vi "Fix merge.vi"(8 "error in (no error)":errorcluster, 11 "Control-Client in":refnum<class "Control-Client.lvclass">) -> (0 "error out":errorcluster, 3 "Control-Client out":refnum<class "Control-Client.lvclass">)   [LabVIEW 2019, in "Control-Client.lvclass"]
uses:
  Control-Client.lvclass
  Experiments/Experiment_merged/Experiment_merged.lvclass
  C:/Dev/TRANCON/Classes/Experiments/Experiment.lvclass
  Control-Client.lvclass/Control-Client.ctl
  Experiments/Experiment.lvclass
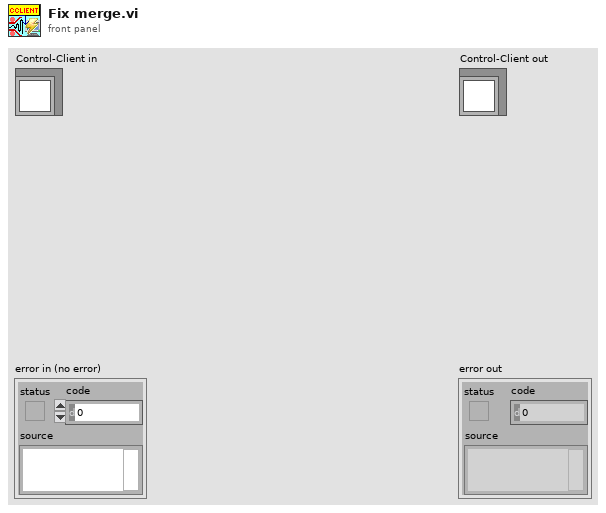
[diagram p1: front panel]
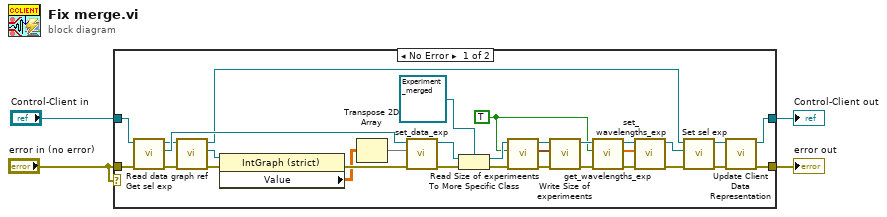
[diagram p0: block diagram]
diagram:
  n1 = case shown="No Error" "error in (no error)" {
    selector: "error in (no error)" -> [_ w37]
    tunnel: [w35 w37] -> w4
    tunnel: [w34 w36] -> w2
    tunnel: "Control-Client in" -> [w29 w36]
    tunnel: "error in (no error)" -> [w28 _]
    frame No Error {
      w7 = TRUE ("Temp")
      n2 = call "Get sel exp.vi"("error in (no error)"=w28, "Control-Client in"=w29) -> ("error out"=w26:errorcluster, "Sel experiment"=w33:refnum<class "Experiment.lvclass">, "Control-Client out"=w27:refnum<class "Control-Client.lvclass">)  [unwired: 7 in]
      n3 = call "Read data graph ref.vi"("error in (no error)"=w26, "Control-Client in"=w27) -> ("error out"=w24:errorcluster, "Exp data graph ref"=w25:refnum<vi>, "Control-Client out"=w32:refnum<class "Control-Client.lvclass">)  [unwired: 7 in]
      n4 = property class="IntGraph (strict)"(reference=w25, error in=w24) -> (error out=w23:errorcluster, "Value"=w22:dbl[][])  [unwired: 1 out]
      n5 = Transpose 2D Array(2D array=w22) -> (transposed array=w21:dbl[][])
      n6 = call "set_data_exp.vi"("error in (no error)"=w23, "Data"=w21, "Experiment.lvclass in"=w33) -> ("error out"=w14:errorcluster, "Experiment.lvclass out"=w20:refnum<class "Experiment.lvclass">)  [unwired: 7 in]
      n7 = To More Specific Class(target class=refnum<class "Experiment_merged.lvclass"> refnum ("Experiment_merged in"), reference=w20, error in=w14) -> (specific class reference=w15:refnum<class "Experiment_merged.lvclass">, error out=w16:errorcluster)
      n8 = call-dynamic "Read Size of experimeents.vi"("error in (no error)"=w16, "Temp"=w7, "Experiment_merged in"=w15) -> ("error out"=w17:errorcluster, "Size of experimeents"=w18:cluster{"X pixels":i32, "Y pixels":i32}[], "Experiment_merged out"=w13:refnum<class "Experiment_merged.lvclass">)  [unwired: 6 in]
      n9 = call-dynamic "Write Size of experimeents.vi"("error in (no error)"=w17, "Size of experimeents"=w18, "Experiment_merged in"=w13) -> ("error out"=w9:errorcluster, "Experiment_merged out"=w8:refnum<class "Experiment_merged.lvclass">)  [unwired: 7 in]
      n10 = call "get_wavelengths_exp.vi"("error in (no error)"=w9, "Temp"=w7, "Experiment.lvclass in"=w8) -> ("error out"=w11:errorcluster, "wavelengths"=w12:dbl[], "Experiment.lvclass out"=w5:refnum<class "Experiment_merged.lvclass">)  [unwired: 6 in]
      n11 = call "set_wavelengths_exp.vi"("error in (no error)"=w11, "wavelengths"=w12, "Experiment.lvclass in"=w5) -> ("error out"=w6:errorcluster, "Experiment.lvclass out"=w10:refnum<class "Experiment_merged.lvclass">)  [unwired: 7 in]
      n12 = call "Set sel exp.vi"("error in (no error)"=w6, "Experiment"=w10, "Control-Client in"=w32) -> ("error out"=w30:errorcluster, "Control-Client out"=w31:refnum<class "Control-Client.lvclass">)  [unwired: 7 in]
      n13 = call "Update Client Data Representation.vi"("error in (no error)"=w30, "Control-Client in"=w31) -> ("error out"=w35:errorcluster, "Control-Client out"=w34:refnum<class "Control-Client.lvclass">)  [unwired: 8 in]
    }
    frame Error {
    }
  }
  "error out" <- w4
  "Control-Client out" <- w2
